vi "Configuration - Read First Analog Out Configuration.vi"(8 "error in":errorcluster) -> (0 "error out":errorcluster, 1 "Timeout (ms)":i32, 2 "Analog Out Control Port":i32, 3 "Carrier Control Port":i32, 5 "AO - Module Configuration":T1)   [LabVIEW 2017, in "Communications Library.lvlib"]
uses:
  Communications Library.lvlib
  Typedefs/DTACQ Module Configuration--Cluster.ctl
  Typedefs/DTACQ Device Type--Enum.ctl
  Typedefs/Functional Global Variable Action--Enum.ctl
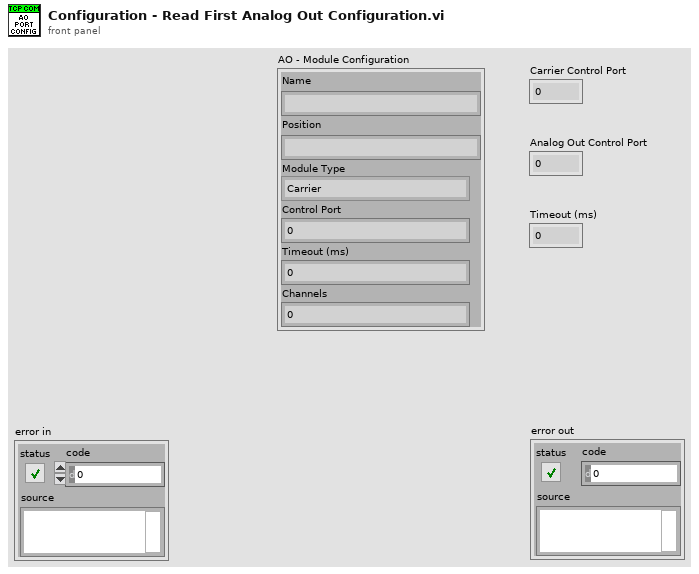
[diagram p1: front panel]
types:
  T1 = typedef "Communications Library.lvlib/DTACQ Module Configuration--Cluster.ctl" = cluster{"Name":string, "Position":string, "Module Type":T2, "Control Port":i32, "Timeout (ms)":i32, "Channels":i32}
  T2 = typedef "Communications Library.lvlib/DTACQ Device Type--Enum.ctl" = enum16{"Carrier", "Analog In Module", "Analog Out Module", "Generic Module"}
  T3 = typedef "Communications Library.lvlib/Functional Global Variable Action--Enum.ctl" = enum16{"Initialise", "Write Module Config", "Write Carrier Config", "Read"}
  T4 = typedef "Communications Library.lvlib/DTACQ Module Carrier Configuration--Cluster.ctl" = cluster{"Name":string, "IP":string, "Control Port":i32, "Timeout (ms)":i32, "Continuous Capture Port (Multiplexed)":i32, "Start HIL Shot Port":i32, "AWG Upload Port (Multiplexed)":i32, "Download Captured Data Port (Multiplexed)":i32, "Module Slots":i32, "Module Configurations":T1[]}
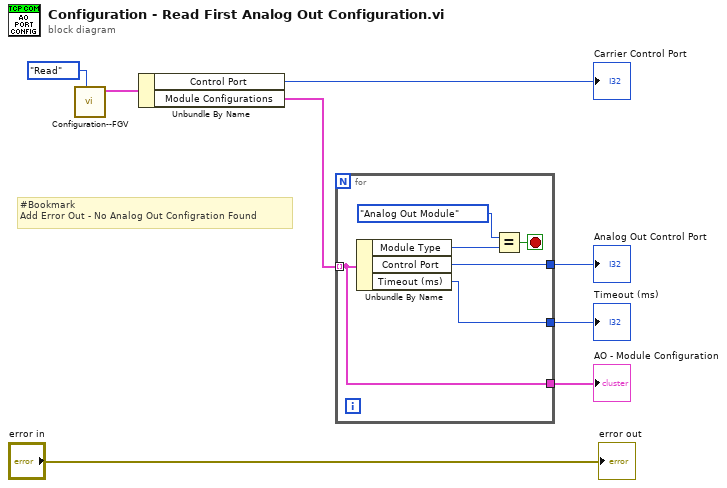
[diagram p0: block diagram]
diagram:
  # "#Bookmark\nAdd Error Out - No Analog Out Configration Found"
  n1 = call "Configuration--FGV.vi"("Functional Global Action"=Functional_Global_Variable_Action--Enum."Read") -> ("Carrier Configuration Out"=w8:T4)  [unwired: 9 in, 1 out]
  n2 = Unbundle By Name(w8) -> ("Control Port"=→"Carrier Control Port":i32, "Module Configurations"=w6:T1[])
  n3 = for {
    tunnel: w6 -> [w9] mode=indexing
    tunnel: [w11] -> w5
    tunnel: [w10] -> w3
    tunnel: [w9] -> w2
    stop <- w12 stop-if-true
    n4 = Unbundle By Name(w9) -> ("Module Type"=w14:T2, "Control Port"=w11:i32, "Timeout (ms)"=w10:i32)
    n5 = Equal?(x=DTACQ_Device_Type--Enum."Analog Out Module", y=w14) -> (x = y?=w12:bool)
  }
  "Analog Out Control Port" <- w5
  "Timeout (ms)" <- w3
  "AO - Module Configuration" <- w2
  "error out" <- "error in"
